vi "API Proxy - Open and Run All Tests.vi"() -> ()   [LabVIEW 2013]
uses:
  <vilib>/addons/_JKI Toolkits/VI Tester/VI Tester Project API.llb/VI Tester Project API.lvlib
panel:
  in  "application reference":refnum<vi>
  out "error out":errorcluster
  in  "error in (no error)":errorcluster
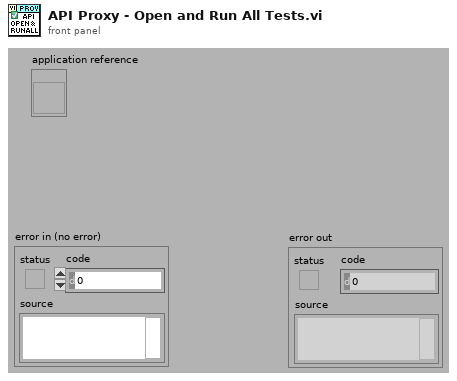
[diagram p1: front panel]
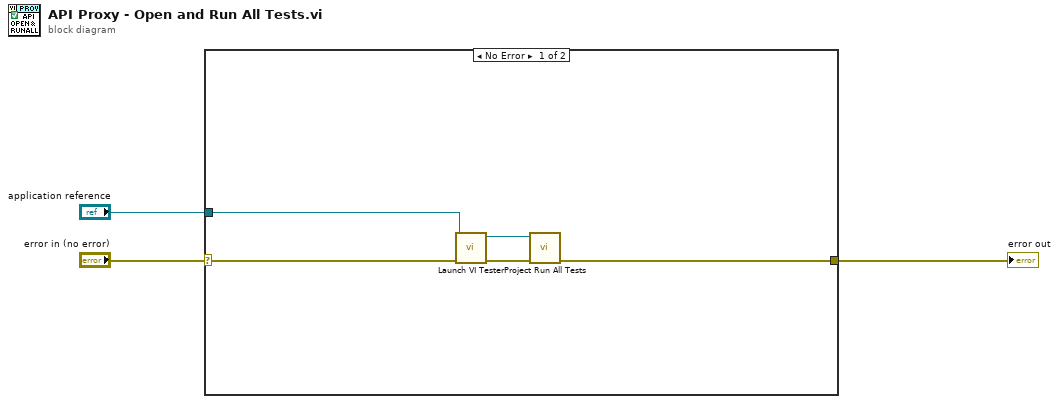
[diagram p0: block diagram]
diagram:
  n1 = case shown="No Error" "error in (no error)" {
    selector: "error in (no error)" -> [w8 w9]
    tunnel: [w6 w9] -> w2
    tunnel: "application reference" -> [w5 _]
    frame No Error {
      n2 = call <vilib>:"Launch VI Tester.vi"("error in (no error)"=w8, "application reference"=w5) -> ("error out"=w7:errorcluster, "VI Tester Ref"=w4:refnum<vi>)  [unwired: 7 in, 1 out]
      n3 = call <vilib>:"Project Run All Tests.vi"("error in (no error)"=w7, "VI Tester reference"=w4) -> ("error out"=w6:errorcluster)  [unwired: 9 in]
    }
    frame Error {
    }
  }
  "error out" <- w2
